vi "Generate Unique ID.vi"(10 "Basename":string, 11 "XML String":string) -> (2 "Unique ID":string)   [LabVIEW 2019, in "EditSVG.lvclass"]
uses:
  EditSVG.lvclass
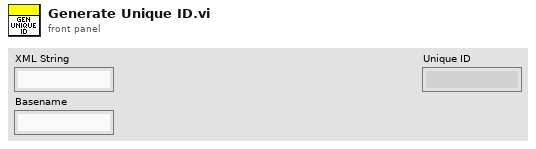
[diagram p1: front panel]
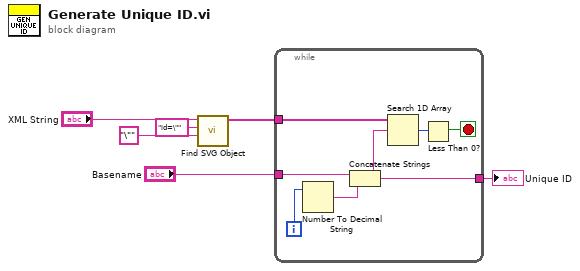
[diagram p0: block diagram]
diagram:
  n1 = call "Find SVG Object.vi"("Ending Delimiter"="\"", "Beginning Delimiter"="id=\"", "XML String"="XML String") -> ("Found Values"=w3:string[])  [unwired: 6 in, 2 out]
  n2 = while {
    tunnel: w3 -> [w10]
    tunnel: "Basename" -> [w13]
    tunnel: [w7] -> w1
    i -> [w12]
    stop <- w8 stop-if-true
    n3 = Number To Decimal String(number=w12) -> (decimal integer string=w11:string)  [unwired: 1 in]
    n4 = Concatenate Strings(w13, w11) -> (w7:string)
    n5 = Search 1D Array(1D array=w10, element=w7) -> (index of element=w9:i32)  [unwired: 1 in]
    n6 = Less Than 0?(x=w9) -> (x < 0?=w8:bool)
  }
  "Unique ID" <- w1
